vi "Test Process Restart.vi"(8 "error in (no error)":errorcluster, 11 "Process Test In":refnum<class "Process Dev Test.lvclass">) -> (0 "error out":errorcluster, 3 "Process Test Out":refnum<class "Process Dev Test.lvclass">)   [LabVIEW 2020, in "Process Dev Test.lvclass"]
uses:
  Process Dev Test.lvclass
  C:/Program Files (x86)/National Instruments/LabVIEW 2020/vi.lib/Astemes/LUnit/Test Case.lvclass
  source/Framework/Process/Public/Lifecycle/Lifecycle State.ctl
  source/Framework Test Suite/Mock Error Handler/Mock Error Handler.lvclass
  C:/Git/triarc-framework/source/Framework/Error Handler Interface/Error Handler Interface.lvclass
  source/Framework/Process/Process.lvclass
  source/Framework/Process/Process.lvclass/Process.ctl
  <vilib>/Astemes/LUnit/Test Case.lvclass/Test Case.ctl
  <vilib>/Astemes/LUnit/LUnit Assertion Result.lvclass/LUnit Assertion Result.ctl
  <vilib>/Astemes/LUnit/LUnit Test Case Result.lvclass/LUnit Test Case Result.ctl
  <vilib>/Astemes/LUnit/LUnit Method Result.lvclass/LUnit Method Result.ctl
  source/Framework/Process/Protected/Messaging/Enqueue Message.vi
  source/Framework/Process/Public/Lifecycle/Get Lifecycle State.vi
  source/Framework/Process/Private/SubVIs/Wait for finish.vi
  source/Framework/Process/Private/SubVIs/Set Lifecycle State.vi
  <vilib>/Astemes/LUnit/Set Assertion Type.vi
  <vilib>/Astemes/LUnit/Palette/Pass.vi
  <vilib>/Astemes/LUnit/Palette/Fail.vi
  source/Framework/Process/Private/SubVIs/Handle Debug Data.vi
  <vilib>/Utility/error.llb/Clear Errors.vi
  <vilib>/Astemes/LUnit/LUnit Write Assertion Type.vi
  <vilib>/Astemes/LUnit/Add test result.vi
  <vilib>/Astemes/LUnit/LUnit Write Passed.vi
  <vilib>/Astemes/LUnit/LUnit Write Message.vi
  <vilib>/Astemes/LUnit/LUnit Write Description.vi
  source/Framework/Logging/Log Debug.vi
  <vilib>/AdvancedString/1D String Array to Delimited String.vi
  <vilib>/Utility/High Resolution Relative Seconds.vi
  <vilib>/Astemes/LUnit/LUnit Record Assertion Result.vi
  <vilib>/Astemes/LUnit/LUnit Aggregate Assertion Results.vi
  <vilib>/Astemes/LUnit/Assertion Result/LUnit Read Status.vi
  <vilib>/Astemes/LUnit/LUnit Read Message.vi
  <vilib>/Astemes/LUnit/LUnit Read Description.vi
  <vilib>/Astemes/LUnit/Method Result/LUnit Merge Status.vi
  <vilib>/Astemes/LUnit/LUnit Concatenate result strings.vi
  <vilib>/Utility/error.llb/Error Cluster From Error Code.vi
  source/Framework/Process/Public/Read Name.vi
  <vilib>/Astemes/LUnit/LUnit Assertion Result.lvclass
  <vilib>/Astemes/LUnit/Test Case.lvclass
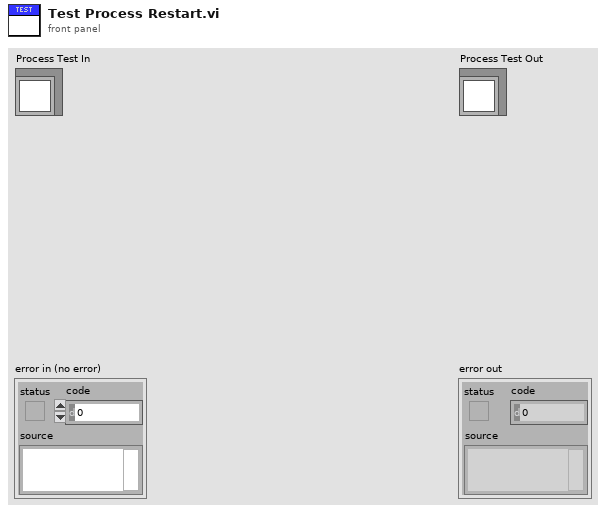
[diagram p1: front panel]
types:
  T1 = typedef "Process.lvclass/Lifecycle State.ctl" = enum16{"Uninitialized", "Initialized", "Started", "Running", "Stopped", "Finished"}
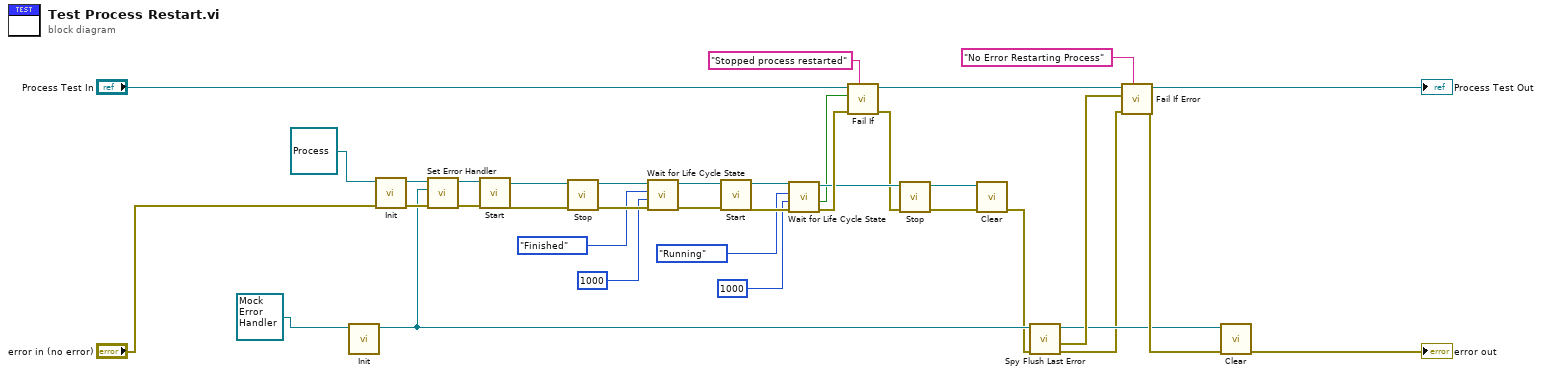
[diagram p0: block diagram]
diagram:
  n1 = call-dynamic "Init.vi"("Mock Error Handler In"=refnum<class "Mock Error Handler.lvclass"> refnum ("Mock Error Handler.lvclass")) -> ("Mock Error Handler Out"=w10:refnum<class "Mock Error Handler.lvclass">)  [unwired: 9 in, 1 out]
  n2 = call-dynamic "Init.vi"("error in (no error)"="error in (no error)", "Process In"=refnum<class "Process.lvclass"> refnum) -> ("error out"=w35:errorcluster, "Process Out"=w16:refnum<class "Process.lvclass">)  [unwired: 8 in]
  n3 = call "Set Error Handler.vi"("error in (no error)"=w35, "Error Handler"=w10, "Process In"=w16) -> ("error out"=w17:errorcluster, "Process Out"=w15:refnum<class "Process.lvclass">)  [unwired: 7 in]
  n4 = call "Start.vi"("error in (no error)"=w17, "Process In"=w15) -> ("error out"=w36:errorcluster, "Process Out"=w37:refnum<class "Process.lvclass">)  [unwired: 7 in, 1 out]
  n5 = call "Stop.vi"("error in (no error)"=w36, "Process In"=w37) -> ("error out"=w30:errorcluster, "Process Out"=w28:refnum<class "Process.lvclass">)  [unwired: 7 in, 1 out]
  n6 = call "Wait for Life Cycle State.vi"("error in (no error)"=w30, "timeout in ms (-1)"=1000, "Lifecycle State"=Lifecycle_State."Finished", "Process In"=w28) -> ("error out"=w29:errorcluster, "Process Out"=w27:refnum<class "Process.lvclass">)  [unwired: 5 in, 1 out]
  n7 = call "Start.vi"("error in (no error)"=w29, "Process In"=w27) -> ("error out"=w33:errorcluster, "Process Out"=w23:refnum<class "Process.lvclass">)  [unwired: 7 in, 1 out]
  n8 = call "Wait for Life Cycle State.vi"("error in (no error)"=w33, "timeout in ms (-1)"=1000, "Lifecycle State"=Lifecycle_State."Running", "Process In"=w23) -> ("error out"=w24:errorcluster, "timed out?"=w18:bool, "Process Out"=w22:refnum<class "Process.lvclass">)  [unwired: 5 in]
  n9 = call <vilib>:"Fail If.vi"("Description"="Stopped process restarted", "error in (no error)"=w24, "Fail?"=w18, "LUnit Test Case In"="Process Test In") -> ("error out"=w19:errorcluster, "LUnit Test Case Out"=w13:refnum<class "Process Dev Test.lvclass">)  [unwired: 6 in]
  n10 = call "Stop.vi"("error in (no error)"=w19, "Process In"=w22) -> ("error out"=w31:errorcluster, "Process Out"=w32:refnum<class "Process.lvclass">)  [unwired: 7 in, 1 out]
  n11 = call-dynamic "Clear.vi"("error in (no error)"=w31, "Process In"=w32) -> ("error out"=w6:errorcluster)  [unwired: 9 in]
  n12 = call "Spy Flush Last Error.vi"("error in (no error)"=w6, "Mock Error Handler In"=w10) -> ("error out"=w5:errorcluster, "Error"=w11:errorcluster, "Mock Error Handler Out"=w7:refnum<class "Mock Error Handler.lvclass">)  [unwired: 7 in]
  n13 = call <vilib>:"Fail If Error.vi"("Description"="No Error Restarting Process", "error in (no error)"=w5, "Assert error"=w11, "LUnit Test Case In"=w13) -> ("error out"=w9:errorcluster, "LUnit Test Case Out"=→"Process Test Out":refnum<class "Process Dev Test.lvclass">)  [unwired: 6 in]
  n14 = call-dynamic "Clear.vi"("error in (no error)"=w9, "Mock Process In"=w7) -> ("error out"=→"error out":errorcluster)  [unwired: 9 in]
